vi "LVClass_HasoSlopes Write HasoSlopes.vi"(8 "error in (no error)":errorcluster, 10 "HasoSlopes":i32, 11 "HasoSlopes in":refnum<class "HasoSlopes.lvclass">) -> (0 "error out":errorcluster, 3 "HasoSlopes out":refnum<class "HasoSlopes.lvclass">)   [LabVIEW 2020, in "HasoSlopes.lvclass"]
uses:
  HasoSlopes.lvclass
  Handle creation.ctl
  HasoSlopes.lvclass/HasoSlopes.ctl
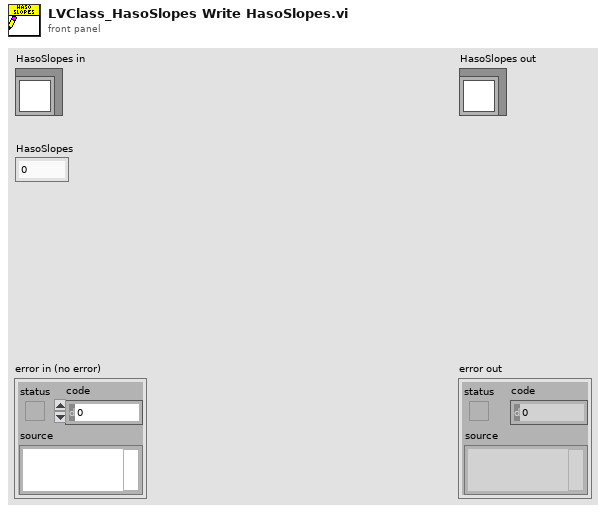
[diagram p1: front panel]
types:
  T1 = typedef "Handle creation.ctl" = enum16{"By ctor", "By write function"}
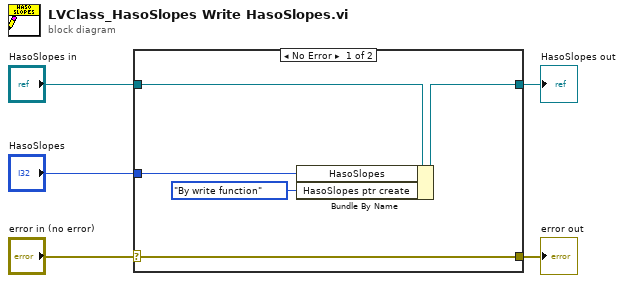
[diagram p0: block diagram]
diagram:
  n1 = case shown="No Error" "error in (no error)" {
    selector: "error in (no error)" -> [w10 w11]
    tunnel: [w10 w11] -> w4
    tunnel: [w8 w12] -> w2
    tunnel: "HasoSlopes in" -> [w9 w12]
    tunnel: "HasoSlopes" -> [w7 _]
    frame No Error {
      n2 = Bundle By Name(cluster=w9, "HasoSlopes"=w7, "HasoSlopes ptr create"=Handle_creation."By write function") -> (w8:refnum<class "HasoSlopes.lvclass">)
    }
    frame Error {
    }
  }
  "error out" <- w4
  "HasoSlopes out" <- w2
